vi "SPD.DCR Meas Const T.vi"(5 "Continue":refnum<vi>, 6 "Temperature index":i32, 7 "Progress":refnum<vi>, 8 "Error In":errorcluster, 10 "DCRParams":T1, 11 "SPD.Stand Ctrl in":T2 {"spdDeviceSession"."hidSPD.Sturtup Values"."HV_bias" format="%#_6p, V"; "spdDeviceSession"."hidSPD.Sturtup Values"."TSet" format="%#_6p, DegC"; "spdDeviceSession"."hidSPD.Controller"."HV_bias" format="%#_6p, V"; "spdDeviceSession"."hidSPD.Controller"."TSet" format="%#_6p, DegC"}) -> (0 "Error Out":errorcluster, 1 "pass":bool, 2 "Report":string, 3 "SPD.Stand Ctrl out":T2 {"spdDeviceSession"."hidSPD.Sturtup Values"."HV_bias" format="%#_6p, V"; "spdDeviceSession"."hidSPD.Sturtup Values"."TSet" format="%#_6p, DegC"; "spdDeviceSession"."hidSPD.Controller"."HV_bias" format="%#_6p, V"; "spdDeviceSession"."hidSPD.Controller"."TSet" format="%#_6p, DegC"})   [LabVIEW 2018]
uses:
  typedefs/SPD.Stand Ctrl.ctl
  Instruments/SPD HID Interface/hidSPDLibForLabView/LibVIs/hidSPD Controls/hidSPD Device Session.ctl
  Instruments/SPD HID Interface/hidSPDLibForLabView/LibVIs/hidSPD Controls/hidSPD Controller.ctl
  Instruments/SPD HID Interface/hidSPDLibForLabView/LibVIs/hidSPD Controls/hidSPD SPD Type.ctl
  Instruments/KC705 DevBoard/typedefs/DevB.Session.ctl
  Instruments/KeySight 53230A/typedefs/FreqC.Session.ctl
  Instruments/KeySight 8164B/KeySight 8164B LAN InstrLib/typedefs/KeySight 8164B control.ctl
  Instruments/LeCroy SDA830/typedefs/LeCroy.Session.ctl
  typedefs/SPD.Events.ctl
  ConfigFile/SPD.Config File ctrl.ctl
  <vilib>/Utility/config.llb/Config Data RefNum.ctl
  typedefs/SPD.Meas Result.ctl
  typedefs/SPD.Queues.ctl
  typedefs/SPD.Stand state.ctl
  typedefs/SPD.DCR Test Params.ctl
  Instruments/KeySight 8164B/KeySight 8164B LAN InstrLib.lvlib
  <vilib>/Utility/config.llb/NI_LVConfig.lvlib
  Instruments/SPD HID Interface/hidSPDLibForLabView/hidSPDLibForLabView.lvlib
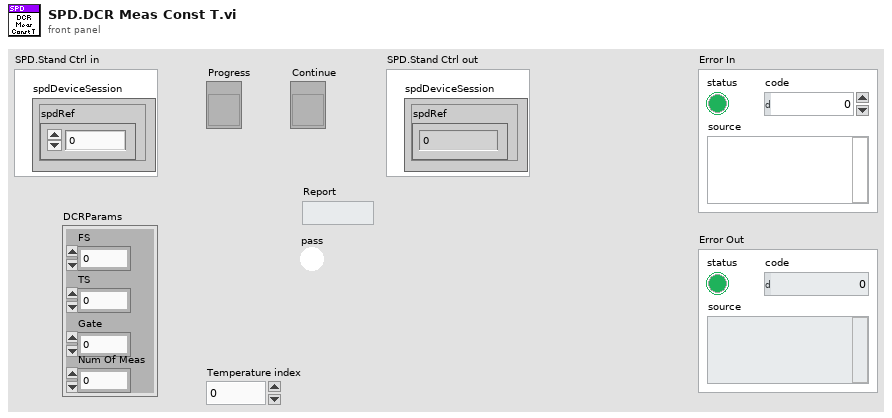
[diagram p1: front panel]
types:
  T1 = typedef "SPD.DCR Test Params.ctl" = cluster{"FS":i32, "TS":i32, "Gate":dbl, "Num Of Meas":i32}
  T2 = typedef "SPD.Stand Ctrl.ctl" = cluster{"spdDeviceSession":T3, "DevBSession":T6, "FreqCSession":T7, "8164BSession":T8, "LeCroySession":T9, "Events":T10, "configFile":T11, "SPD.Result":T13, "SPD.Queues":T14, "Console":refnum<vi>}
  T3 = typedef "hidSPDLibForLabView.lvlib/hidSPD Device Session.ctl" = cluster{"spdRef":u64, "connected":bool, "spdName":string, "hidSPD.Controller":T4, "hidSPD.Sturtup Values":T4, "SPD Type":T5}
  T4 = typedef "hidSPDLibForLabView.lvlib/hidSPD Controller.ctl" = cluster{"TSet":sgl, "HV_bias":sgl, "DDS_stb_code":u16}
  T5 = typedef "hidSPDLibForLabView.lvlib/hidSPD SPD Type.ctl" = enum16{"Free Run", "Gate"}
  T6 = typedef "DevB.Session.ctl" = cluster{"DevBRef":refnum<visa-resource-name>, "connected":bool}
  T7 = typedef "FreqC.Session.ctl" = cluster{"FreqCRef":refnum<visa-resource-name>, "timeout":dbl, "Gate":dbl, "connected":bool}
  T8 = typedef "KeySight 8164B LAN InstrLib.lvlib/KeySight 8164B control.ctl" = cluster{"Connection ID":refnum<k5>, "Connected":bool, "Info":string, "Slots Info":string[]}
  T9 = typedef "LeCroy.Session.ctl" = cluster{"LeCroySession":refnum<visa-resource-name>, "connected":bool}
  T10 = typedef "SPD.Events.ctl" = cluster{"DCRTest":refnum<user-event>, "Stop":refnum<user-event>}
  T11 = typedef "SPD.Config File ctrl.ctl" = cluster{"configFile ref":T12, "configFile path":path, "equipmentFile ref":T12}
  T12 = typedef "NI_LVConfig.lvlib/Config Data RefNum.ctl" = refnum<k1>
  T13 = typedef "SPD.Meas Result.ctl" = cluster{"HV_Bias":dbl[][][], "Stb_code":dbl[], "Temprature":dbl[], "Data":dbl[][][][], "DateTime":string}
  T14 = typedef "SPD.Queues.ctl" = cluster{"state queue":refnum<queue>}
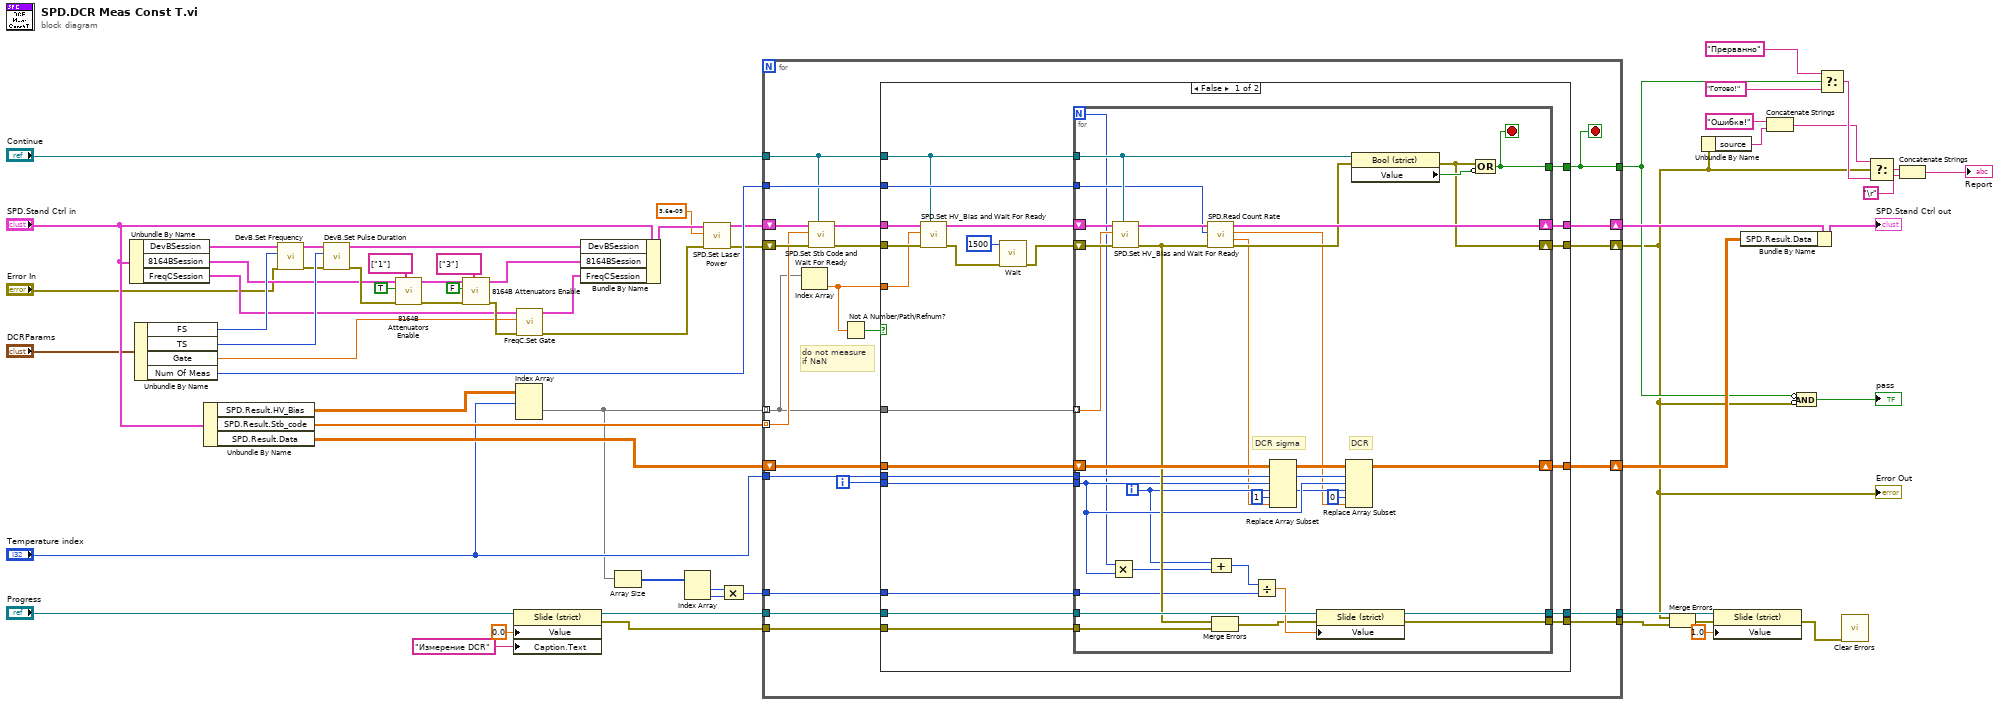
[diagram p0: block diagram]
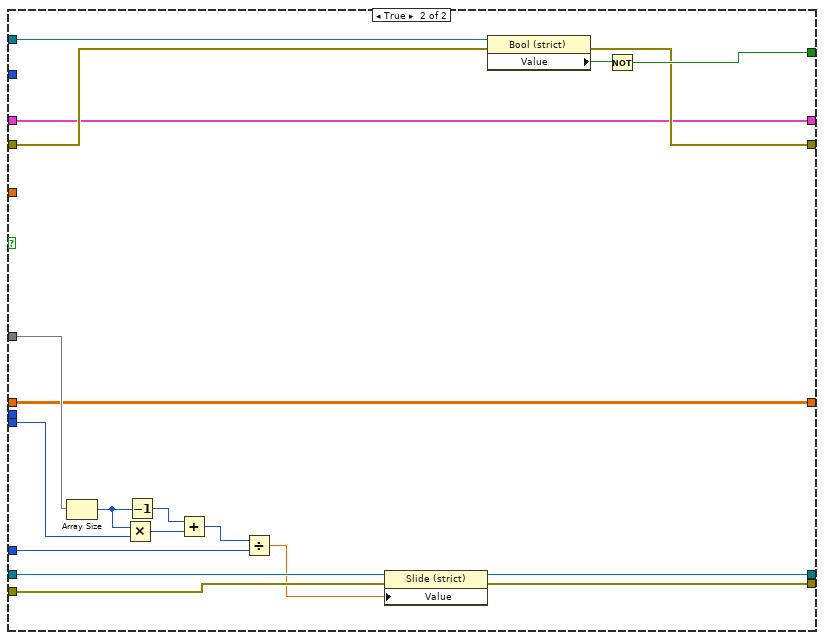
[diagram p2: hidden frame]
diagram:
  n1 = Unbundle By Name("SPD.Stand Ctrl in") -> ("DevBSession"=w53:T6, "8164BSession"=w40:T8, "FreqCSession"=w39:T7)
  n2 = Unbundle By Name("DCRParams") -> ("FS"=w51:i32, "TS"=w50:i32, "Gate"=w34:dbl, "Num Of Meas"=w31:i32)
  n3 = Unbundle By Name("SPD.Stand Ctrl in") -> ("SPD.Result.HV_Bias"=w54:dbl[][][], "SPD.Result.Stb_code"=w55:dbl[], "SPD.Result.Data"=w30:dbl[][][][])
  n4 = call "DevB.Set Frequency.vi"("error in (no error)"="Error In", "Frequency"=w51, "DevB Session in"=w53) -> ("error out"=w49:errorcluster, "DevB Session out"=w52:T6)  [unwired: 7 in]
  n5 = call "DevB.Set Pulse Duration.vi"("error in (no error)"=w49, "Pulse Duration"=w50, "DevB Session in"=w52) -> ("error out"=w42:errorcluster, "DevB Session out"=w38:T6)  [unwired: 7 in]
  n6 = call "8164B Attenuators Enable.vi"("Slots"=string[] ["1"], "error in"=w42, "Enable"=TRUE, "KeySight 8164B control in"=w40) -> ("error out"=w46:errorcluster, "KeySight 8164B control out"=w45:T8)  [unwired: 6 in]
  n7 = call "8164B Attenuators Enable.vi"("Slots"=string[] ["3"], "error in"=w46, "Enable"=FALSE, "KeySight 8164B control in"=w45) -> ("error out"=w41:errorcluster, "KeySight 8164B control out"=w37:T8)  [unwired: 6 in]
  n8 = property class="Slide (strict)"(reference="Progress", "Value"=0.0, "Caption.Text"="Измерение DCR") -> (reference out=w15:refnum<vi>, error out=w13:errorcluster)  [unwired: 1 in]
  n9 = Index Array(array=w54, index (dim 0)="Temperature index") -> (element=w7:dbl[][])  [unwired: 2 in]
  n10 = call "FreqC.Set Gate.vi"("error In"=w41, "Gate, sec"=w34, "FreqC Session in"=w39) -> ("error out"=w4:errorcluster, "FreqC Session out"=w36:T7)  [unwired: 7 in]
  n11 = Bundle By Name(cluster="SPD.Stand Ctrl in", "DevBSession"=w38, "8164BSession"=w37, "FreqCSession"=w36) -> (w5:T2)
  n12 = Array Size(array=w7) -> (size(s)=w29:i32[])
  n13 = Index Array(array=w29) -> (element #1=w28:i32, element #2=w27:i32)  [unwired: 2 in]
  n14 = call "SPD.Set Laser Power.vi"("Error In"=w4, "Pset"=3.6e-09, "SPD.Stand Ctrl in"=w5) -> ("Error Out"=w3:errorcluster, "SPD.Stand Ctrl out"=w2:T2)  [unwired: 7 in]
  n15 = Compound Arithmetic op=MULTIPLY(w28, w27) -> (w59:i32)
  n16 = for {
    shift-right: [w83] -> w60
    shift-left: w30 -> [w85]
    tunnel: w7 -> [w68] mode=indexing
    tunnel: w55 -> [w79] mode=indexing
    shift-right: [w84] -> w63
    shift-left: w2 -> [w81]
    shift-right: [w82] -> w6
    shift-left: w3 -> [w80]
    tunnel: "Continue" -> [w69]
    tunnel: "Temperature index" -> [w78]
    tunnel: [w76] -> w9
    tunnel: w15 -> [w75]
    tunnel: w59 -> [w74]
    tunnel: [w73] -> w58
    tunnel: w31 -> [w72]
    tunnel: w13 -> [w67]
    tunnel: [w66] -> w11
    i -> [w77]
    stop <- w76 stop-if-true
    # "do not measure\nif NaN"
    n17 = Index Array(array=w68) -> (element=w64:dbl)  [unwired: 1 in]
    n18 = call "SPD.Set Stb Code and Wait For Ready.vi"("Continue"=w69, "Error In"=w80, "Strobe code"=w79, "SPD.Stand Ctrl in"=w81) -> ("Error Out"=w70:errorcluster, "SPD.Stand Ctrl out"=w71:T2)  [unwired: 6 in]
    n19 = Not A Number/Path/Refnum?(number/path/refnum=w64) -> (NaN/Path/Refnum?=w65:bool)
    n20 = case shown="False" w65 {
      tunnel: w85 -> [w107 w140]
      tunnel: [w106 w153] -> w84
      tunnel: [w105 w140] -> w83
      tunnel: [w104 w154] -> w82
      tunnel: w78 -> [w103 _]
      tunnel: w77 -> [w102 w147]
      tunnel: [w101 w156] -> w76
      tunnel: w75 -> [w100 w151]
      tunnel: w74 -> [w99 w142]
      tunnel: [w98 w149] -> w73
      tunnel: w72 -> [w97 _]
      tunnel: w71 -> [w96 w153]
      tunnel: w70 -> [w95 w155]
      tunnel: w69 -> [w93 w158]
      tunnel: w68 -> [w92 w148]
      tunnel: w64 -> [w91 _]
      tunnel: w67 -> [w90 w152]
      tunnel: [w89 w150] -> w66
      frame False {
        n21 = call "SPD.Set HV_Bias and Wait For Ready.vi"("Continue"=w93, "Error In"=w95, "HV_Bias"=w91, "SPD.Stand Ctrl in"=w96) -> ("Error Out"=w88:errorcluster, "SPD.Stand Ctrl out"=w94:T2)  [unwired: 6 in]
        n22 = call "Wait.vi"("error in (no error)"=w88, "milliseconds to wait"=u32 1500) -> ("error out"=w87:errorcluster)  [unwired: 9 in]
        n23 = for {
          N -> [w111]
          tunnel: w92 -> [w133] mode=indexing
          shift-right: [w120] -> w105
          shift-left: w107 -> [w139]
          shift-right: [w138] -> w106
          shift-left: w94 -> [w136]
          shift-right: [w130] -> w104
          shift-left: w87 -> [w134]
          tunnel: w93 -> [w132]
          tunnel: w103 -> [w119]
          tunnel: w102 -> [w118]
          tunnel: [w129] -> w101
          tunnel: w100 -> [w128]
          tunnel: w99 -> [w125]
          tunnel: [w123] -> w98
          tunnel: w97 -> [w113]
          tunnel: w90 -> [w109]
          tunnel: [w108] -> w89
          i -> [w117]
          stop <- w129 stop-if-true
          # "DCR"
          # "DCR sigma"
          n24 = Multiply(x=w111, y=w118) -> (x*y=w112:i32)
          n25 = call "SPD.Set HV_Bias and Wait For Ready.vi"("Continue"=w132, "Error In"=w134, "HV_Bias"=w133, "SPD.Stand Ctrl in"=w136) -> ("Error Out"=w127:errorcluster, "SPD.Stand Ctrl out"=w135:T2)  [unwired: 6 in]
          n26 = call "SPD.Read Count Rate.vi"("Error In"=w127, "Num of Meas"=w113, "SPD.Stand Ctrl in"=w135) -> ("Error Out"=w137:errorcluster, "Count sigma"=w115:dbl, "Count"=w114:dbl, "SPD.Stand Ctrl out"=w138:T2)  [unwired: 5 in]
          n27 = Compound Arithmetic op=ADD(w117, w112) -> (w126:i32)
          n28 = Merge Errors(w127, w109) -> (w110:errorcluster)
          n29 = Divide(x=w126, y=w125) -> (x/y=w124:dbl)
          n30 = Replace Array Subset(array=w139, new element=w115, index (dim 0)=w119, index (dim 1)=w118, index (dim 2)=w117, index (dim 3)=1 ("disabled index (col)")) -> (w121:dbl[][][][])
          n31 = property class="Slide (strict)"(reference=w128, error in=w110, "Value"=w124) -> (reference out=w123:refnum<vi>, error out=w108:errorcluster)
          n32 = Replace Array Subset(array=w121, new element=w114, index (dim 0)=w119, index (dim 1)=w118, index (dim 2)=w117, index (dim 3)=0 ("disabled index (col)")) -> (w120:dbl[][][][])
          n33 = property class="Bool (strict)"(reference=w132, error in=w137) -> (error out=w130:errorcluster, "Value"=w131:bool)  [unwired: 1 out]
          n34 = Compound Arithmetic op=OR(w130, invert w131) -> (w129:bool)
        }
      }
      frame True {
        n35 = Array Size(array=w148) -> (size(s)=w146:i32)
        n36 = Multiply(x=w146, y=w147) -> (x*y=w144:i32)
        n37 = Decrement(x=w146) -> (x-1=w145:i32)
        n38 = Add(x=w145, y=w144) -> (x+y=w143:i32)
        n39 = Divide(x=w143, y=w142) -> (x/y=w141:dbl)
        n40 = property class="Slide (strict)"(reference=w151, error in=w152, "Value"=w141) -> (reference out=w149:refnum<vi>, error out=w150:errorcluster)
        n41 = property class="Bool (strict)"(reference=w158, error in=w155) -> (error out=w154:errorcluster, "Value"=w157:bool)  [unwired: 1 out]
        n42 = Not(x=w157) -> (.not. x?=w156:bool)
      }
    }
  }
  "Error Out" <- w6
  n43 = Merge Errors(w6, w11) -> (w12:errorcluster)
  n44 = Unbundle By Name(w6) -> ("source"=w22:string)
  n45 = property class="Slide (strict)"(reference=w58, error in=w12, "Value"=1.0) -> (error out=w56:errorcluster)  [unwired: 1 out]
  n46 = Bundle By Name(cluster=w63, "SPD.Result.Data"=w60) -> (→"SPD.Stand Ctrl out":T2)
  n47 = Concatenate Strings("Ошибка!" ("t"), w22) -> (w23:string)
  n48 = Compound Arithmetic op=AND(invert w9, invert w6) -> (→"pass":bool)
  n49 = Select(t="Прерванно" ("Report"), s=w9, f="Готово!") -> (s? t:f=w25:string)
  n50 = call <vilib>:"Clear Errors.vi"("error in (no error)"=w56) -> ()  [unwired: 5 in, 2 out]
  n51 = Select(t=w23, s=w6, f=w25) -> (s? t:f=w20:string)
  n52 = Concatenate Strings(w20, "\r") -> (→"Report":string)
